vi "Remove Panel at Index.vi"(7 "Close Removed (T)":bool=TRUE, 8 "error in (no error)":errorcluster, 9 "2D Index":T1, 11 "2DArrayManager in":refnum<class "2DArrayManager.lvclass">) -> (0 "error out":errorcluster, 1 "Element Removed":bool, 2 "Removed Element":refnum<class "ArrayPanel.lvclass">, 3 "2DArrayManager out":refnum<class "2DArrayManager.lvclass">)   [LabVIEW 2020, in "OOPanel.lvlib" / "2DArrayManager.lvclass"]
uses:
  2DArrayManager.lvclass
  2D Index.ctl
  ArrayPanel/ArrayPanel.lvclass
  2DArrayManager.lvclass/2DArrayManager.ctl
  ArrayPanel/ArrayPanel.lvclass/ArrayPanel.ctl
  OOPanel.lvlib
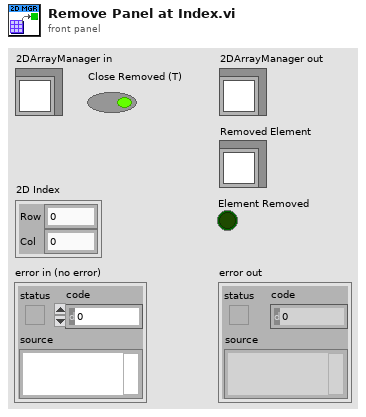
[diagram p1: front panel]
types:
  T1 = typedef "OOPanel.lvlib/2D Index.ctl" = cluster{"Row":i32, "Col":i32}
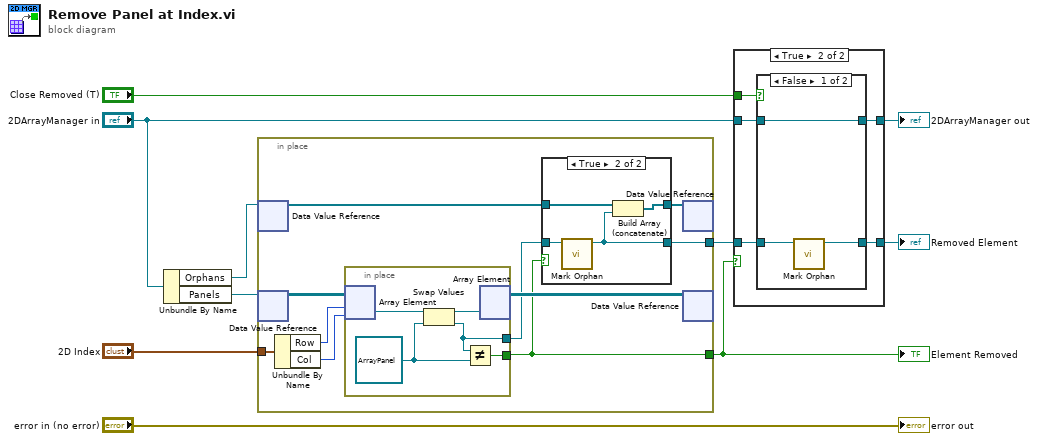
[diagram p0: block diagram]
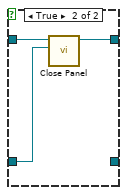
[diagram p3: hidden frame]
diagram:
  n1 = Unbundle By Name("2DArrayManager in") -> ("Orphans"=w9:refnum<data-value>, "Panels"=w8:refnum<data-value>)
  n2 = in-place {
    in-place-border: "2D Index" -> [w19]
    in-place-border: [w14] -> w1
    in-place-border: [w11] -> w3
    n3 = in-place-dvr #1(w9) -> (w15:refnum<class "ArrayPanel.lvclass">[])  [unwired: 1 out]
    n4 = in-place-dvr #2(w8) -> (w20:refnum<class "ArrayPanel.lvclass">[][])  [unwired: 1 out]
    n5 = Unbundle By Name(w19) -> ("Row"=w18:i32, "Col"=w17:i32)
    n6 = in-place {
      in-place-border: [w22] -> w14
      in-place-border: [w21] -> w13
      w23 = refnum<class "ArrayPanel.lvclass"> refnum ("element")
      n7 = in-place-array #3(w20, w18, w17) -> (w25:refnum<class "ArrayPanel.lvclass">)
      n8 = Swap Values(12:w25, 14:w23) -> (1:w24:refnum<class "ArrayPanel.lvclass">, 3:w21:refnum<class "ArrayPanel.lvclass">)  [unwired: 1 in]
      n9 = Not Equal?(x=w21, y=w23) -> (x != y?=w22:bool)
      n10 = in-place-array #3(w24) -> (w16:refnum<class "ArrayPanel.lvclass">[][])  [unwired: 2 out]
    }
    n11 = case shown="True" w14 {
      tunnel: w15 -> [w26 w30]
      tunnel: w13 -> [_ w29]
      tunnel: [w26 w28] -> w12
      tunnel: [_ w27] -> w11
      frame False {
      }
      frame True {
        n12 = call "Mark Orphan.vi"("ArrayPanel in"=w29) -> ("ArrayPanel out"=w27:refnum<class "ArrayPanel.lvclass">)  [unwired: 9 in, 1 out]
        n13 = Build Array (concatenate)(w30, w27) -> (w28:refnum<class "ArrayPanel.lvclass">[])
      }
    }
    n14 = in-place-dvr #1(w12) -> ()  [unwired: 2 out]
    n15 = in-place-dvr #2(w16) -> ()  [unwired: 2 out]
  }
  "Element Removed" <- w1
  n16 = case shown="True" w1 {
    tunnel: w3 -> [_ w36]
    tunnel: [_ w35] -> w2
    tunnel: "Close Removed (T)" -> [_ w34]
    tunnel: "2DArrayManager in" -> [w31 w33]
    tunnel: [w31 w32] -> w6
    frame False {
    }
    frame True {
      n17 = case shown="False" w34 {
        tunnel: w36 -> [w39 w42]
        tunnel: [w38 _] -> w35
        tunnel: w33 -> [w37 w41]
        tunnel: [w37 w40] -> w32
        frame False {
          n18 = call "Mark Orphan.vi"("ArrayPanel in"=w39) -> ("ArrayPanel out"=w38:refnum<class "ArrayPanel.lvclass">)  [unwired: 9 in, 1 out]
        }
        frame True {
          n19 = call "Close Panel.vi"("ArrayPanel"=w42, "2DArrayManager in"=w41) -> ("2DArrayManager out"=w40:refnum<class "2DArrayManager.lvclass">)  [unwired: 8 in, 1 out]
        }
      }
    }
  }
  "2DArrayManager out" <- w6
  "Removed Element" <- w2
  "error out" <- "error in (no error)"
